vi "Scheme.Update Image.vi"(6 "Replace Image":path, 8 "error in":errorcluster, 9 "New Color":u32(colorbox)=14450432, 10 "New Control":path, 11 "Material-Scheme.lvclass":refnum<class "Material-Scheme.lvclass">) -> (0 "error out":errorcluster, 3 "Material-Scheme.lvclass out":refnum<class "Material-Scheme.lvclass">)   [LabVIEW 2021, in "TSC Material Theme.lvlib" / "Material-Scheme.lvclass"]
doc: "Update the image of the buttons\n\n<b>Code Developed By:</b>\nTechnology Service Corporation\nwww.tsc.com/atcs\n\nDeveloper:\nDaniel Coons"
uses:
  Material-Scheme.lvclass
  Material-Scheme.lvclass/Material-Scheme.ctl
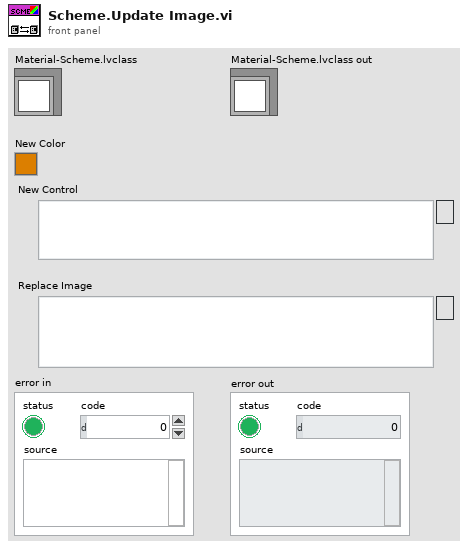
[diagram p1: front panel]
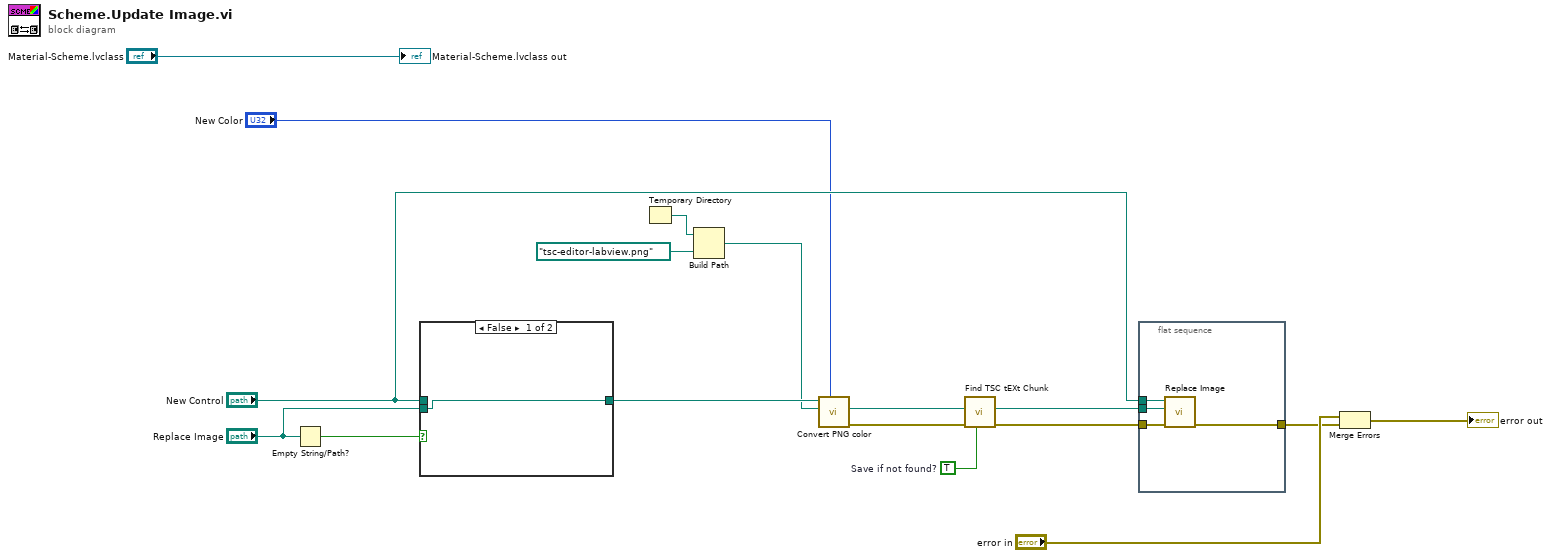
[diagram p0: block diagram]
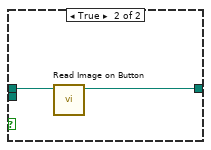
[diagram p2: hidden frame]
diagram:
  w3 = TRUE  # Save if not found?
  n1 = Empty String/Path?(string/path="Replace Image") -> (empty?=w16:bool)
  n2 = case shown="False" w16 {
    tunnel: [w18 w20] -> w10
    tunnel: "New Control" -> [_ w19]
    tunnel: "Replace Image" -> [w18 _]
    frame False {
    }
    frame True {
      n3 = call "Read Image on Button.vi"("File with Button"=w19) -> ("png file out"=w20:path)  [unwired: 9 in, 1 out]
    }
  }
  n4 = Temporary Directory() -> (w9:path)
  n5 = Build Path(base path=w9, name or relative path=path "tsc-editor-labview.png") -> (appended path=w2:path)
  n6 = call "Convert PNG color.vi"("New Color"="New Color", "new file"=w2, "orig file"=w10) -> ("error out"=w6:errorcluster, "new file out"=w4:path)  [unwired: 6 in, 1 out]
  n7 = call "Find TSC tEXt Chunk.vi"("Save if not found?"=w3, "error in"=w6, "file path (use dialog)"=w4) -> ("error out"=w5:errorcluster, "file path dup"=w1:path)  [unwired: 6 in, 1 out]
  n8 = flat-sequence {
    tunnel: "New Control" -> [w24]
    tunnel: w5 -> [w23]
    tunnel: [w22] -> w11
    tunnel: w1 -> [w21]
    frame #0 {
      n9 = call "Replace Image.vi"("error in"=w23, "PNG Image File"=w21, "LabVIEW File with Button"=w24) -> ("error out"=w22:errorcluster)  [unwired: 7 in, 1 out]
    }
  }
  n10 = Merge Errors("error in", w11) -> (→"error out":errorcluster)
  "Material-Scheme.lvclass out" <- "Material-Scheme.lvclass"
